vi "Configure Sweep Trigger.vi"(0 "VISA resource name":refnum<visa-resource-name>, 1 "Point Trigger (1: Immediate)":u16(ring)=1 items=["Bus", "Immediate", "External", "Key", "Timer"], 2 "Enable Continuous Sweep (T:Enable)":bool=TRUE, 5 "Sweep Trigger (1: Immediate)":u16(ring)=1 items=["Bus", "Immediate", "External", "Key", "Timer"], 7 "Trigger Out Polarity (0: Positive)":u16(ring) items=["Positive", "Negative"], 9 "Trigger In Polarity (0: Positive)":u16(ring) items=["Positive", "Negative"], 11 "error in (no error)":errorcluster, 12 "Timer Trigger Period (1 ms)":dbl=0.001) -> (4 "VISA resource name out":refnum<visa-resource-name>, 15 "error out":errorcluster)   [LabVIEW 2011, in "Agilent PSG MXG Series.lvlib"]
doc: "Configures the trigger for list or step sweep."
uses:
  Agilent PSG MXG Series.lvlib
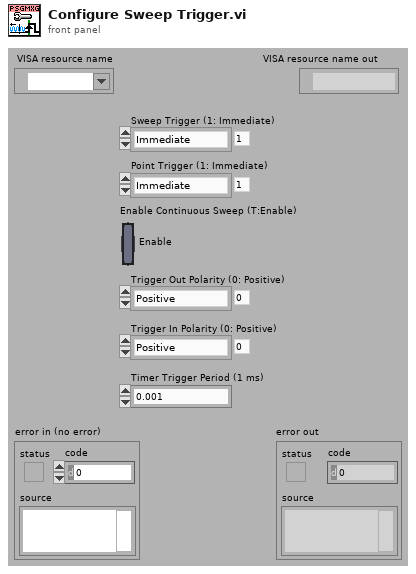
[diagram p1: front panel]
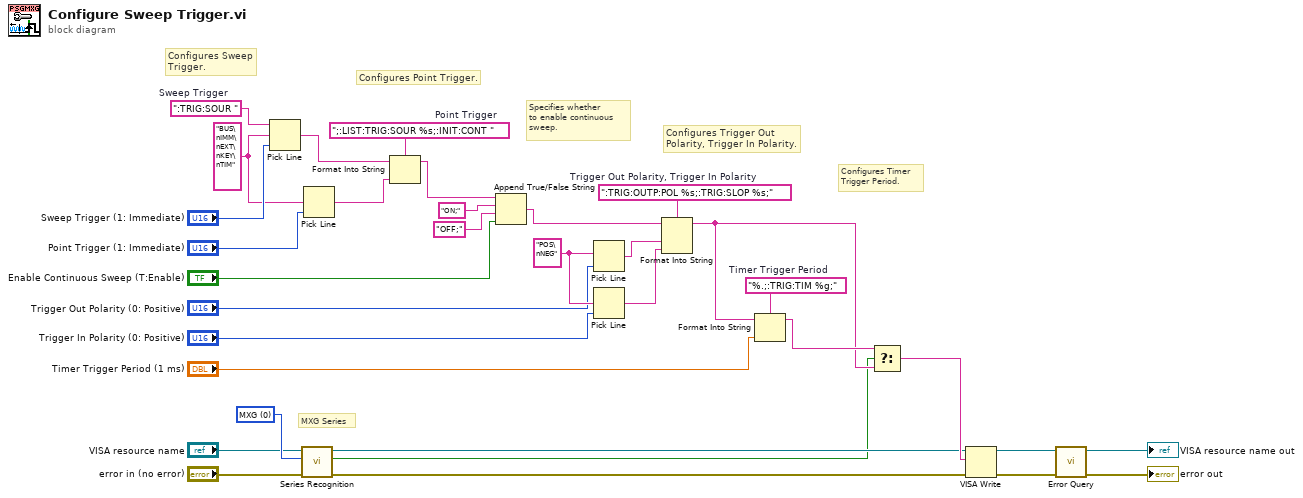
[diagram p0: block diagram]
diagram:
  w8 = u16 0 items=["MXG", "PSG", "PSG-A", "PSG-C", "PSG-D"] ("Series Type (0: MXG)")
  w16 = "%.;:TRIG:TIM %g;"  # Timer Trigger Period
  w20 = "POS\nNEG" ("multi-line string")
  w22 = ":TRIG:OUTP:POL %s;:TRIG:SLOP %s;"  # Trigger Out Polarity, Trigger In Polarity
  w29 = ";:LIST:TRIG:SOUR %s;:INIT:CONT "  # Point Trigger
  w31 = "BUS\nIMM\nEXT\nKEY\nTIM" ("multi-line string")
  w33 = ":TRIG:SOUR "  # Sweep Trigger
  # "Configures Timer\nTrigger Period."
  # "Configures Trigger Out\nPolarity, Trigger In Polarity."
  # "Specifies whether\nto enable continuous\nsweep."
  # "Configures Point Trigger."
  # "Configures Sweep\nTrigger."
  # "MXG Series"
  n1 = Pick Line(string ("")=w33, multi-line string=w31, line index="Sweep Trigger (1: Immediate)") -> (output string=w28:string)
  n2 = call "Series Recognition.vi"("error in (no error)"="error in (no error)", "Series Type (0: MXG)"=w8, "VISA resource name"="VISA resource name") -> ("error out"=w6:errorcluster, "Is Series Correct"=w5:bool, "VISA resource name out"=w7:refnum<visa-resource-name>)  [unwired: 6 in]
  n3 = Pick Line(multi-line string=w31, line index="Point Trigger (1: Immediate)") -> (output string=w27:string)  [unwired: 1 in]
  n4 = Format Into String(format string=w29, initial string=w28, w27) -> (resulting string=w26:string)  [unwired: 1 in, 1 out]
  n5 = Append True/False String(1:"Enable Continuous Sweep (T:Enable)", 2:"OFF;" ("false string"), 3:"ON;" ("true string"), 4:w26) -> (0:w23:string)
  n6 = Pick Line(multi-line string=w20, line index="Trigger Out Polarity (0: Positive)") -> (output string=w21:string)  [unwired: 1 in]
  n7 = Pick Line(multi-line string=w20, line index="Trigger In Polarity (0: Positive)") -> (output string=w17:string)  [unwired: 1 in]
  n8 = Format Into String(format string=w22, initial string=w23, w21, w17) -> (resulting string=w13:string)  [unwired: 1 in, 1 out]
  n9 = Format Into String(format string=w16, initial string=w13, "Timer Trigger Period (1 ms)") -> (resulting string=w14:string)  [unwired: 1 in, 1 out]
  n10 = Select(t=w14, s=w5, f=w13) -> (s? t:f=w12:string)
  n11 = VISA Write(VISA resource name=w7, write buffer=w12, error in (no error)=w6) -> (VISA resource name out=w11:refnum<visa-resource-name>, error out=w10:errorcluster)  [unwired: 1 out]
  n12 = call "Error Query.vi"("error in (no error)"=w10, "VISA resource name"=w11) -> ("error out"=→"error out":errorcluster, "VISA resource name out"=→"VISA resource name out":refnum<visa-resource-name>)  [unwired: 6 in, 2 out]
